vi "Create Quiver.vi"(7 "3D Quiver Property":T5={"General Property"={"Plot Name"="", "Coordinate System"=enum."Cartesian", "Opacity"=0.0}, "Projection Property"={"Draw XY"=FALSE, "Draw YZ"=FALSE, "Draw XZ"=FALSE}, "Plot Property"={"Line Style"=enum."None", "Line Width"=0.0, "Line Color"=0, "Antialiasing"=FALSE, "Color Ramp Cluster"={"Color Ramp Style"=enum."None", "Color Ramp Array"=[16711934, 393471, 57855, 4390754, 16449346, 16744722, 16711680], "Color Ramp Index"=[45, 91, 133, 175, 219, 255], "Interpolate?"=FALSE, "Logarithm?"=FALSE}}, "Quiver Property"={"Quvier Mode"=enum."Quiver", "Quiver Size"=0.0, "Quiver Length"=0.0}}, 8 "error in (no error)":errorcluster, 9 "Actual Transform In":T1, 10 "Plot Representation In":T3, 11 "Plot Object In":refnum<vi>) -> (0 "error out":errorcluster, 1 "Actual Transform Out":T1, 2 "Plot Representation Out":T3, 3 "Plot Object Out":refnum<vi>, 4 "Quiver Object Out":refnum<vi>)   [LabVIEW 2020, in "3D Quiver.lvclass"]
uses:
  <vilib>/Math Plots/3D Math Plots/3D Quiver/3D Quiver/3D Quiver.lvclass
  <vilib>/Math Plots/3D Math Plots/3D Quiver/3D Quiver/Typedef/3D Quiver Property.ctl
  <vilib>/Math Plots/3D Math Plots/3D Plot/3D Plot/Typedef/Line Type.ctl
  <vilib>/Math Plots/3D Math Plots/3D Plot/3D Plot/Typedef/Color Ramp Cluster.ctl
  <vilib>/Math Plots/3D Math Plots/3D Plot/3D Plot/Typedef/Plot Representation.ctl
  <vilib>/Math Plots/3D Math Plots/3D Plot/3D Plot/Typedef/Range Clusters.ctl
  <vilib>/Math Plots/3D Math Plots/3D Plot/3D Plot/Typedef/Mesh Data.ctl
  <vilib>/Math Plots/3D Math Plots/3D Plot/3D Plot/Typedef/Actual Transform.ctl
  <vilib>/picture/3D Picture Control/NI_3D Picture Control.lvlib
  <vilib>/Math Plots/3D Math Plots/3D Plot/3D Plot/3D Plot.lvclass
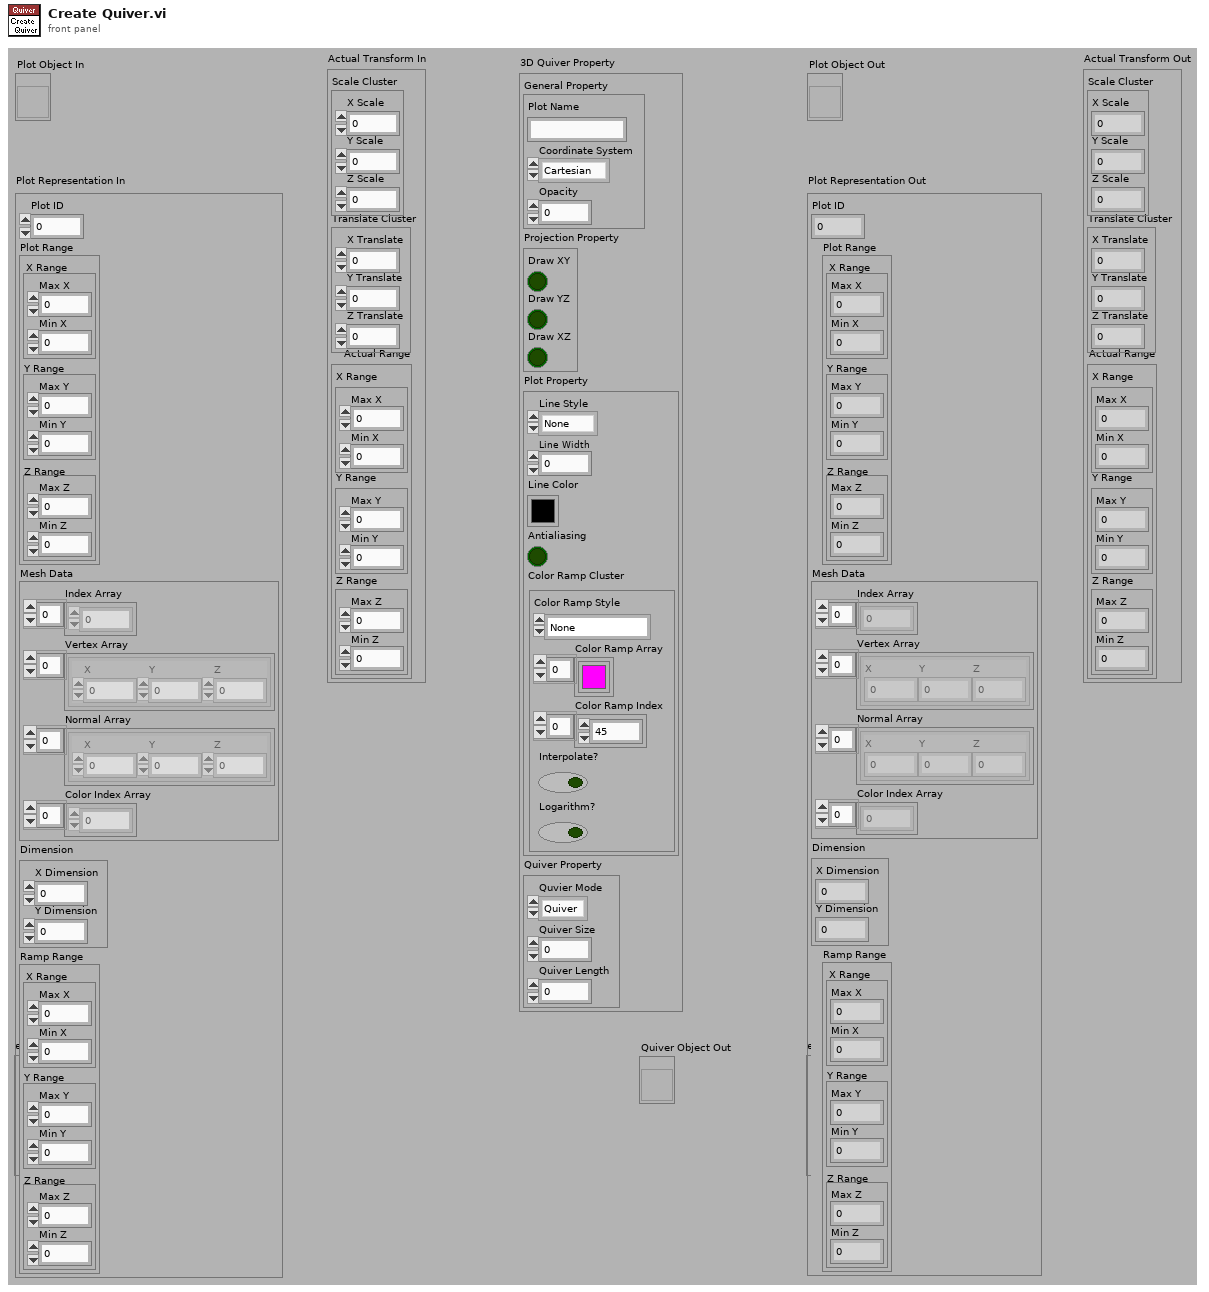
[diagram p1: front panel]
types:
  T1 = typedef "3D Plot.lvclass/Actual Transform.ctl" = cluster{"Scale Cluster":cluster{"X Scale":sgl, "Y Scale":sgl, "Z Scale":sgl}, "Translate Cluster":cluster{"X Translate":sgl, "Y Translate":sgl, "Z Translate":sgl}, "Actual Range":T2}
  T2 = typedef "3D Plot.lvclass/Range Clusters.ctl" = cluster{"X Range":cluster{"Max X":sgl, "Min X":sgl}, "Y Range":cluster{"Max Y":sgl, "Min Y":sgl}, "Z Range":cluster{"Max Z":sgl, "Min Z":sgl}}
  T3 = typedef "3D Plot.lvclass/Plot Representation.ctl" = cluster{"Plot ID":i32, "Plot Range":T2, "Mesh Data":T4, "Dimension":cluster{"X Dimension":i32, "Y Dimension":i32}, "Ramp Range":T2}
  T4 = typedef "3D Plot.lvclass/Mesh Data.ctl" = cluster{"Index Array":u32[], "Vertex Array":cluster{"X":sgl, "Y":sgl, "Z":sgl}[], "Normal Array":cluster{"X":sgl, "Y":sgl, "Z":sgl}[], "Color Index Array":i32[]}
  T5 = typedef "3D Quiver.lvclass/3D Quiver Property.ctl" = cluster{"General Property":cluster{"Plot Name":string, "Coordinate System":enum16{"Cartesian", "Cylindrical", "Spherical"}, "Opacity":sgl}, "Projection Property":cluster{"Draw XY":bool, "Draw YZ":bool, "Draw XZ":bool}, "Plot Property":cluster{"Line Style":T6, "Line Width":sgl, "Line Color":u32, "Antialiasing":bool, "Color Ramp Cluster":T7}, "Quiver Property":cluster{"Quvier Mode":enum16{"Quiver", "Quiver with surface"}, "Quiver Size":sgl, "Quiver Length":sgl}}
  T6 = typedef "3D Plot.lvclass/Line Type.ctl" = enum16{"None", "Solid", "Dash", "Dot", "Dash Dot"}
  T7 = typedef "3D Plot.lvclass/Color Ramp Cluster.ctl" = cluster{"Color Ramp Style":enum16{"None", "Shaded", "Color spectrum", "Grey scale", "Custom"}, "Color Ramp Array":u32[], "Color Ramp Index":i32[], "Interpolate?":bool, "Logarithm?":bool}
  T8 = enum16{"Overall", "Per Primitive", "Per Vertex", "Binding Off"}
  T9 = enum16{"Points", "Lines", "Line Strip", "Line Loop", "Triangles", "Triangle Strip", "Triangle Fan", "Quads", "Quad Strip", "Polygon"}
  T10 = cluster{"X Scale":sgl, "Y Scale":sgl, "Z Scale":sgl}
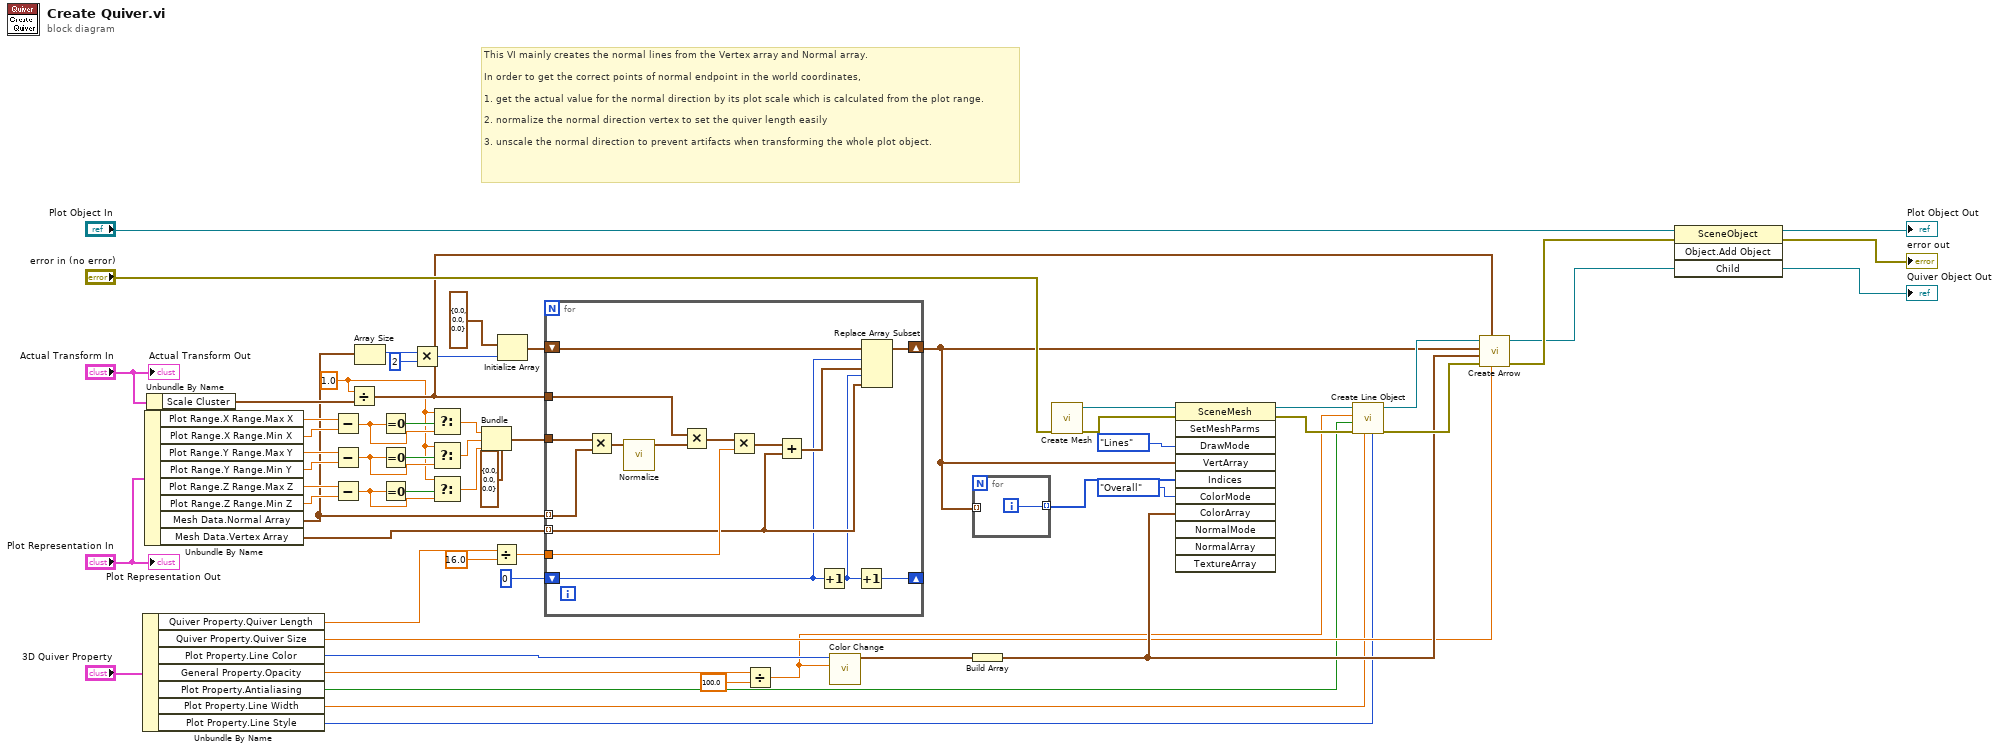
[diagram p0: block diagram]
diagram:
  w1 = sgl 1.0
  # "This VI mainly creates the normal lines from the Vertex array and Normal array.\n\nIn order to get the correct points of normal endpoint in the world coordinates,\n\n1. get the actual value for the normal direction by its plot scale which is calculated from the plot range.\n\n2. normalize the normal direction vertex to set the quiver length easily\n\n3. unscale the normal direction to prevent artifacts when transforming the whole plot object."
  n1 = Unbundle By Name("3D Quiver Property") -> ("Quiver Property.Quiver Length"=w11:sgl, "Quiver Property.Quiver Size"=w35:sgl, "Plot Property.Line Color"=w41:u32, "General Property.Opacity"=w24:sgl, "Plot Property.Antialiasing"=w27:bool, "Plot Property.Line Width"=w26:sgl, "Plot Property.Line Style"=w28:T6)
  n2 = Unbundle By Name("Plot Representation In") -> ("Plot Range.X Range.Max X"=w34:sgl, "Plot Range.X Range.Min X"=w33:sgl, "Plot Range.Y Range.Max Y"=w32:sgl, "Plot Range.Y Range.Min Y"=w31:sgl, "Plot Range.Z Range.Max Z"=w30:sgl, "Plot Range.Z Range.Min Z"=w29:sgl, "Mesh Data.Normal Array"=w16:cluster{"X":sgl, "Y":sgl, "Z":sgl}[], "Mesh Data.Vertex Array"=w21:cluster{"X":sgl, "Y":sgl, "Z":sgl}[])
  n3 = Unbundle By Name("Actual Transform In") -> ("Scale Cluster"=w43:T10)
  n4 = Subtract(x=w34, y=w33) -> (x-y=w5:sgl)
  n5 = Subtract(x=w32, y=w31) -> (x-y=w4:sgl)
  n6 = Subtract(x=w30, y=w29) -> (x-y=w9:sgl)
  n7 = Divide(x=w1, y=w43) -> (x/y=w42:T10)
  n8 = Array Size(array=w16) -> (size(s)=w15:i32)
  n9 = Equal To 0?(x=w5) -> (x = 0?=w6:bool)
  n10 = Equal To 0?(x=w4) -> (x = 0?=w7:bool)
  n11 = Equal To 0?(x=w9) -> (x = 0?=w10:bool)
  n12 = Multiply(x=w15, y=2) -> (x*y=w14:i32)
  n13 = Select(t=w1, s=w6, f=w5) -> (s? t:f=w3:sgl)
  n14 = Select(t=w1, s=w7, f=w4) -> (s? t:f=w2:sgl)
  n15 = Select(t=w1, s=w10, f=w9) -> (s? t:f=w8:sgl)
  n16 = Bundle(cluster=cluster{"X":sgl, "Y":sgl, "Z":sgl} {"X"=0.0, "Y"=0.0, "Z"=0.0} ("Vector"), "X"=w3, "Y"=w2, "Z"=w8) -> (w61:cluster{"X":sgl, "Y":sgl, "Z":sgl})
  n17 = Divide(x=w11, y=sgl 16.0) -> (x/y=w46:sgl)
  n18 = Initialize Array(cluster{"X":sgl, "Y":sgl, "Z":sgl} {"X"=0.0, "Y"=0.0, "Z"=0.0} ("3D Point"), w14) -> (w18:cluster{"X":sgl, "Y":sgl, "Z":sgl}[])
  n19 = for {
    tunnel: w16 -> [w75] mode=indexing
    tunnel: w21 -> [w65] mode=indexing
    tunnel: w61 -> [w76]
    tunnel: w46 -> [w73]
    shift-right: [w67] -> w19
    shift-left: w18 -> [w68]
    tunnel: w42 -> [w69]
    shift-right: [w64] -> _
    shift-left: 0 ("y") -> [w62]
    n20 = Multiply(x=w76, y=w75) -> (x*y=w74:cluster{"X":sgl, "Y":sgl, "Z":sgl})
    n21 = call <vilib>:"Normalize.vi"("Vector"=w74) -> ("Normalized Vector"=w71:cluster{"X":sgl, "Y":sgl, "Z":sgl})  [unwired: 10 out]
    n22 = Multiply(x=w69, y=w71) -> (x*y=w70:cluster{sgl, sgl, sgl})
    n23 = Multiply(x=w70, y=w73) -> (x*y=w72:cluster{sgl, sgl, sgl})
    n24 = Add(x=w72, y=w65) -> (x+y=w66:cluster{sgl, sgl, sgl})
    n25 = Increment(x=w62) -> (x+1=w63:i32)
    n26 = Increment(x=w63) -> (x+1=w64:i32)
    n27 = Replace Array Subset(array=w68, new element #1=w66, index #1=w62, new element #2=w65, index #2=w63) -> (w67:cluster{"X":sgl, "Y":sgl, "Z":sgl}[])
  }
  n28 = Divide(x=w24, y=sgl 100.0) -> (x/y=w23:sgl)
  n29 = call <vilib>:"Color Change.vi"("Alpha"=w23, "Color"=w41) -> ("RGBA"=w56:cluster{"R":sgl, "G":sgl, "B":sgl, "A":sgl})  [unwired: 9 out]
  n30 = for {
    tunnel: [w77] -> w20 mode=indexing
    tunnel: w19 -> [_] mode=indexing
    i -> [w77]
  }
  n31 = Build Array(w56) -> (w36:cluster{"R":sgl, "G":sgl, "B":sgl, "A":sgl}[])
  n32 = call <vilib>:"Create Mesh.vi"("error in (no error)"="error in (no error)") -> ("error out"=w55:errorcluster, "New Mesh Refnum"=w58:refnum<vi>)  [unwired: 9 out]
  n33 = invoke class="SceneMesh" method="SetMeshParms"(reference=w58, error in=w55, "DrawMode"=T9."Lines" ("Draw Mode"), "VertArray"=w19, "Indices"=w20, "ColorMode"=T8."Overall" ("Color Binding Mode"), "ColorArray"=w36) -> (reference out=w38:refnum<vi>, error out=w37:errorcluster)  [unwired: 4 in, 9 out]
  n34 = call <vilib>:"Create Line Object.vi"("Line Style"=w28, "Line Width"=w26, "error in (no error)"=w37, "Antialiasing"=w27, "Alpha"=w23, "Mesh Ref In"=w38) -> ("error out"=w39:errorcluster, "Object Ref Out"=w40:refnum<vi>)  [unwired: 4 out]
  n35 = call <vilib>:"Create Arrow.vi"("Quiver Size"=w35, "Scale"=w42, "error in (no error)"=w39, "Color Array"=w36, "Normal Vertex"=w19, "Quiver Object In"=w40) -> ("error out"=w45:errorcluster, "Quiver Object Out"=w44:refnum<vi>)  [unwired: 1 in, 3 out]
  n36 = invoke class="SceneObject" method="Object.Add Object"(reference="Plot Object In", error in=w45, "Child"=w44) -> (reference out=→"Plot Object Out":refnum<vi>, error out=→"error out":errorcluster, "Child"=→"Quiver Object Out":refnum<vi>)  [unwired: 1 in, 1 out]
  "Plot Representation Out" <- "Plot Representation In"
  "Actual Transform Out" <- "Actual Transform In"
